vi "TestExecuteWriteWhenVisibleSubscription_NoUpdate.vi"(8 "error in (no error)":errorcluster, 11 "TestCase in":refnum<class "TestSubscriptionPolicy.lvclass">) -> (0 "error out":errorcluster, 3 "TestCase out":refnum<class "TestSubscriptionPolicy.lvclass">)   [LabVIEW 2017, in "TestSubscriptionPolicy.lvclass"]
uses:
  TestSubscriptionPolicy.lvclass
  IMediator/ISubscriptionPolicy/ISubscriptionPolicy.lvclass/ISubscriptionPolicy.ctl
  WriteWhenVisibleSubscription/WriteWhenVisibleSubscription.lvclass
  C:/Git/mva-framework/Framework/IMediator/ISubscriptionPolicy/ISubscriptionPolicy.lvclass
  Transport/TerminalBinding/TerminalBinding.lvclass
  C:/Git/mva-framework/Framework/IMediator/ITransport/ITransport.lvclass
  IMediator/ISubscriptionPolicy/ISubscriptionPolicy.lvclass
panel:
  in  "Numeric":dbl
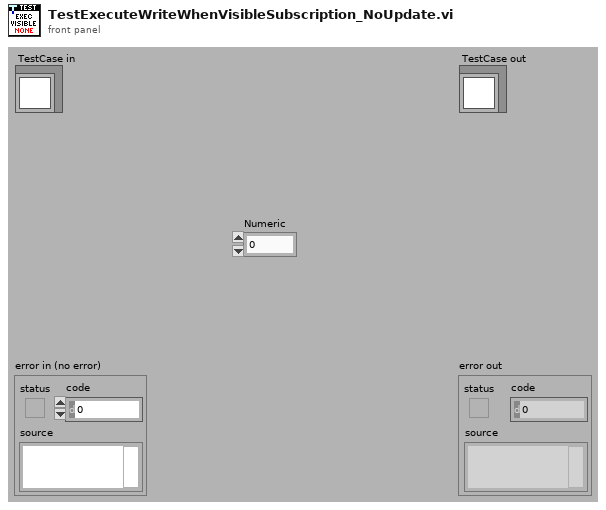
[diagram p1: front panel]
types:
  T1 = typedef "IMediator.lvlib/ISubscriptionPolicy.lvclass/ISubscriptionPolicy Reference.ctl" = refnum<data-value>
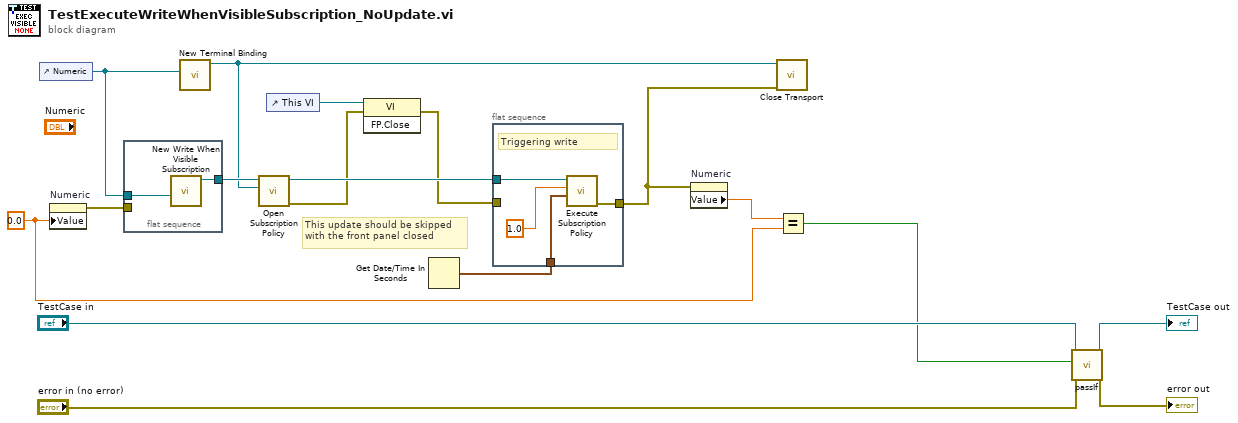
[diagram p0: block diagram]
diagram:
  w1 = 0.0 ("Numeric")
  # "This update should be skipped\nwith the front panel closed"
  n1 = control-ref of="Numeric"() -> (w4:refnum<vi>)
  n2 = property on="Numeric" class="DigNum (strict)"("Value"=w1) -> (error out=w6:errorcluster)  [unwired: 2 in, 1 out]
  n3 = flat-sequence {
    tunnel: [w19] -> w13
    tunnel: w6 -> [_]
    tunnel: w4 -> [w18]
    frame #0 {
      n4 = call "New Write When Visible Subscription.vi"("Ctl Refnum"=w18) -> ("WriteWhenVisibleSubscription Out"=w19:refnum<class "WriteWhenVisibleSubscription.lvclass">)  [unwired: 10 in]
    }
  }
  n5 = call "New Terminal Binding.vi"("Ctl Refnum"=w4) -> ("TerminalBinding"=w11:refnum<class "TerminalBinding.lvclass">)  [unwired: 9 in, 1 out]
  n6 = call "Open Subscription Policy.vi"("Transport"=w11, "SubscriptionPolicy"=w13) -> ("error out"=w8:errorcluster, "Subscription Policy"=w12:T1)  [unwired: 8 in]
  n7 = control-ref of="This VI"() -> (w9:refnum<vi>)
  n8 = invoke class="VI" method="FP.Close"(reference=w9, error in=w8) -> (error out=w7:errorcluster)  [unwired: 1 in, 2 out]
  n9 = Get Date/Time In Seconds() -> (seconds since 1Jan1904=w10:timestamp)
  n10 = flat-sequence {
    tunnel: w12 -> [w23]
    tunnel: w10 -> [w22]
    tunnel: [w21] -> w2
    tunnel: w7 -> [_]
    frame #0 {
      # "Triggering write"
      n11 = call "Execute Subscription Policy.vi"("Publish Time"=w22, "New Topic Value"=1.0, "Subscription Policy"=w23) -> ("error out (Unsubscribe?)"=w21:errorcluster)  [unwired: 8 in]
    }
  }
  n12 = property on="Numeric" class="DigNum (strict)"(error in=w2) -> ("Value"=w5:dbl)  [unwired: 1 in, 2 out]
  n13 = call-dynamic "Close Transport.vi"("error in (no error)"=w2, "ITransport in"=w11) -> ()  [unwired: 9 in, 1 out]
  n14 = Equal?(x=w5, y=w1) -> (x = y?=w3:bool)
  n15 = call-dynamic "passIf.vi"("error in (no error)"="error in (no error)", "pass"=w3, "TestCase in"="TestCase in") -> ("error out"=→"error out":errorcluster, "TestCase out"=→"TestCase out":refnum<class "TestSubscriptionPolicy.lvclass">)  [unwired: 7 in]
